vi "play_AFMss_integral_trajTrack_extend.vi"() -> ()   [LabVIEW 2015]
uses:
  controls/controlParams_tracktraj.ctl
  <vilib>/userdefined/High Color/nirio_resource_hc.ctl
  <vilib>/Utility/file.llb/Read From Spreadsheet File (DBL).vi
  <vilib>/FPGAPlugInAG/cRIO-9082/niLvFpga_Open_cRIO-9082.vi
  <vilib>/rvi/interface/common/dynamic/niFpgaDynamicAddResources.vi
  <vilib>/FPGAPlugInAG/Dynamic/niLvFpga_Reset_Dynamic.vi
  <vilib>/rvi/interface/common/niFpgaWaitOnOcc.vi
  <vilib>/Utility/error.llb/Error Cluster From Error Code.vi
  <vilib>/rvi/errors/niLvFpgaAdjustHostInterfaceError.vi
  <vilib>/FPGAPlugInAG/Dynamic/niLvFpga_Run_Dynamic.vi
  <vilib>/Utility/file.llb/Write To Spreadsheet File (DBL).vi
  <vilib>/FPGAPlugInAG/Dynamic/niLvFpga_Close_Dynamic.vi
  <vilib>/rvi/interface/nirviOpenFPGA/nirviOpenFPGA.xnode
  FPGA Bitfiles/AFMsssinglematri_FPGATargetSPARTA_AFMsscontrolDela_G9MTOUg9BHM.lvbitx
  <vilib>/rvi/interface/nirviMethod/nirviMethod.xnode
  <vilib>/rvi/interface/nirviReadWriteControl/nirviReadWriteControl.xnode
  <vilib>/rvi/interface/nirviCloseFPGA/nirviCloseFPGA.xnode
  <vilib>/FPGAPlugInAG/Dynamic/niLvFpga_ConfigureFifo_Dynamic.vi
  <vilib>/rvi/errors/niLvFpgaMergeErrorWithErrorCode.vi
  <vilib>/rvi/interface/Simulation/niFpgaSimulationCallBeginRW.vi
  <vilib>/FPGAPlugInAG/Dynamic/niLvFpga_ReadFifo_Dynamic.vi
  <vilib>/FPGAPlugInAG/Dynamic/niLvFpga_WriteFifo_Dynamic.vi
  NiFpgaLv.dll
panel:
  in  "N":i32
  in  "control_data_path":path=path "C:/Users/arnold/Documents/MATLAB/AFM_SS/data/ref_traj_track.csv"
  out "Actual Depth":u32
  out "YK TO":bool
  out "UK TO":bool
  out "yk":sgl
  out "loop ticks benchmark":sgl
  out "Xd_out(k+1)":sgl[](array[numeric])
  in  "Cluster":T1={"umax"=3.0, "y_ref(k)"=0.0, "Ki"=0.0, "y(k) (from plant)"=0.0, "ND"=0, "NS"=0, "u_Kx_ref(k)"=0.0} {"u_Kx_ref(k)" format="%#_13g"; "Ki" format="%#_13g"; "y_ref(k)" format="%#_13g"; "umax" format="%#_13g"}
  out "Unstable Traj":bool
  out "Control Loop Done":bool
  out "Elements Remaining":u32
  out "Arow10":sgl[](array[numeric])=[0.0, 0.0, 0.0, 0.0, 0.0, 0.0, 0.90156674, 0.0, 0.0]
  out "Arow9":sgl[](array[numeric])=[0.0, 0.0, 0.0, 0.0, 0.0, 0.0, 0.90156674, 0.0, 0.0]
  out "Arow8":sgl[](array[numeric])=[0.0, 0.0, 0.0, 0.0, 0.0, 0.0, 0.90156674, 0.0, 0.0]
  out "elements left":i32=1
  in  "reference traj path":path=path "C:/Users/arnold/Documents/MATLAB/AFM_SS/data/ref_traj_track.csv"
  in  "outputData BOTH":path=path "C:/Users/arnold/Documents/MATLAB/AFM_SS/data/exp01outputBOTH.csv"
  out "x+1":i32
  out "ND":i32
  out "NS":i32
  in  "Tab Control":enum32{"Custom Params", "Loaded Params"}(tab)
  in  "Nbar":dbl=1.253469179440319 format="%#_13g"
  in  "Ki":dbl=0.125346917944 format="%#_13g"
  out "Nbar":dbl=1.253469179440319 format="%#_13g"
  out "Ki":dbl=0.125346917944 format="%#_13g"
  out "ref":dbl format="%#_13g"
  in  "SettleTicks":i32=10
  in  "Stop":bool=TRUE
  out "y iter":i32
  out "u iter":i32
  out "size(s) 5":i32
  out "size(s)":i32
  out "Arow7":sgl[](array[numeric])=[0.0, 0.0, 0.0, 0.0, 0.0, 0.0, 0.90156674, 0.0, 0.0]
  out "Arow6":sgl[](array[numeric])=[0.0, 0.0, 0.0, 0.0, -0.0009308535, 0.009943728, 1.1488396, 0.0, 0.0]
  out "Arow5":sgl[](array[numeric])=[0.0, 0.0, 0.0, 0.0, 0.99437284, 0.09308535, 3.730764, 0.0, 0.0]
  out "Arow4":sgl[](array[numeric])=[0.0, 0.0, -0.16696692, 0.97962993, 29.579603, 1.2871753, 39.36298, 0.0, 0.0]
  out "Arow3":sgl[](array[numeric])=[0.0, 0.0, 0.97962993, 0.16696692, 2.4679432, 0.11174757, 2.9240768, 0.0, 0.0]
  out "K_in 2":sgl[](array[numeric])=[-0.023819132, 0.00010408472, 0.0, 0.0, 0.0, 0.0, 0.0, 0.0, 0.0]
  out "K_in":sgl[](array[numeric])=[-0.023819132, 0.00010408472, 0.0, 0.0, 0.0, 0.0, 0.0, 0.0, 0.0]
  out "Arow2_in":sgl[](array[numeric])=[-0.21879435, 0.97156703, 5.4823804, 0.59487915, 7.8694544, 0.30187303, 8.202156, 0.0, 0.0]
  out "Arow1_in":sgl[](array[numeric])=[0.97156703, 0.21879435, 0.7281903, 0.07828272, 1.117765, 0.037789278, 0.6448556, 0.0, 0.0]
  out "C_in":sgl[](array[numeric])=[-8.076578e-08, -5.6617e-09, 2.3556278e-05, -6.9169624e-07, -0.005420799, 0.00037984832, -0.012524399, 0.0, 0.0]
  out "L_in":sgl[](array[numeric])=[-2254.4756, -17288.861, -3886.0125, -24956.67, -705.887, -3987.6506, -7.2153935, 0.0, 0.0]
  out "Bz_in":sgl[](array[numeric])=[-0.0016434871, -0.020676594, -0.010679029, -0.20639984, -0.030792456, -1.3413852, -0.02736353, 0.0, 0.0]
  in  "Iters":i32=25
  in  "Cont Run (F)":bool=TRUE
  in  "ymax":dbl=4.0 format="%#_13g"
  in  "umax":dbl=1.0 format="%#_13g"
  in  "TsTicks":i32=1600
  # "Manually define Parameters"
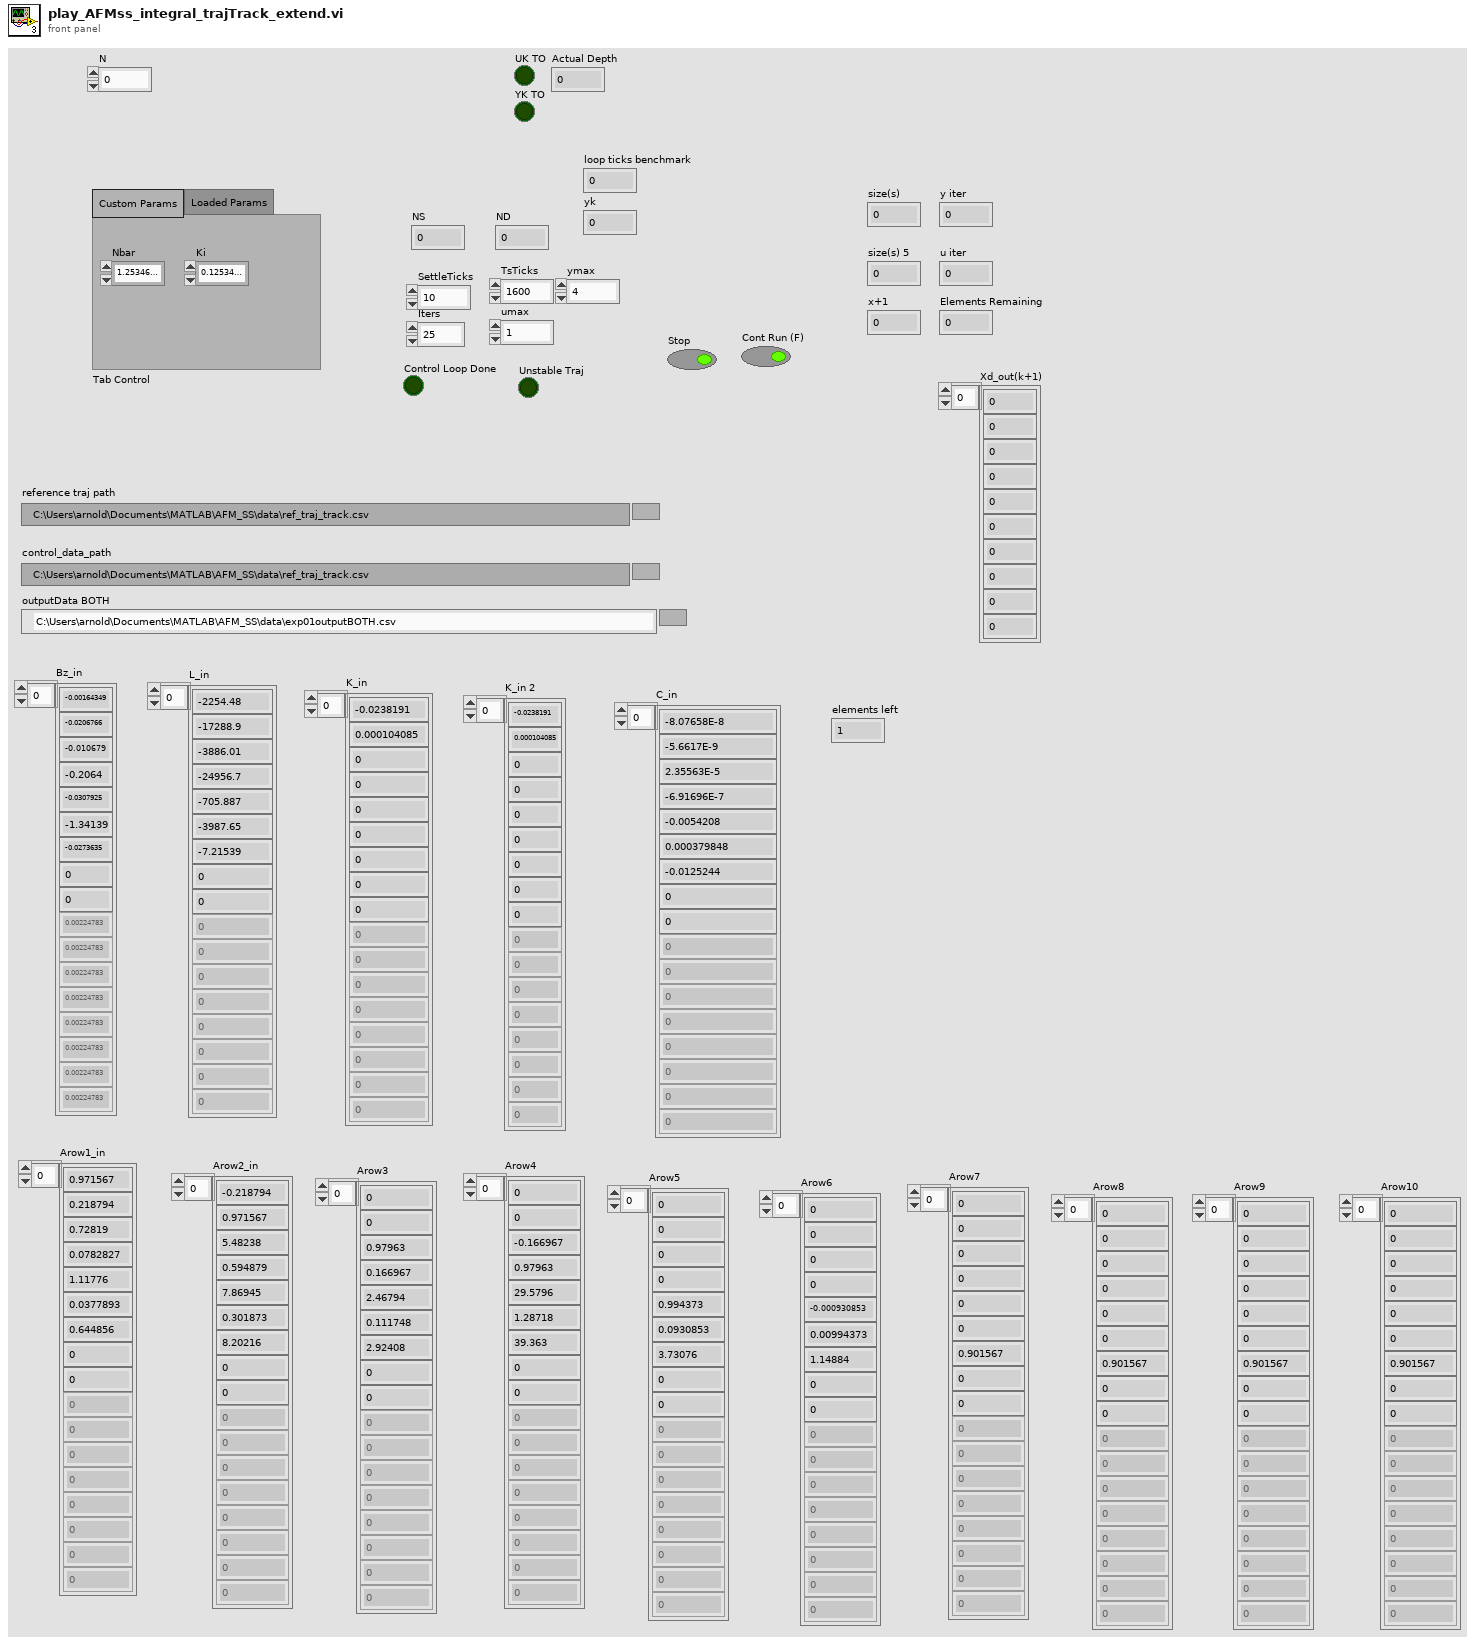
[diagram p1: front panel]
types:
  T1 = typedef "controlParams_tracktraj.ctl" = cluster{"umax":sgl, "y_ref(k)":sgl, "Ki":sgl, "y(k) (from plant)":sgl, "ND":i16, "NS":i16, "u_Kx_ref(k)":sgl}
  T2 = typedef "nirio_resource_hc.ctl" = tag
  T3 = typedef "ControlParams.ctl" = cluster{"NS":i32, "ND":i32, "Nbar":dbl, "Ki":dbl, "ref":dbl}
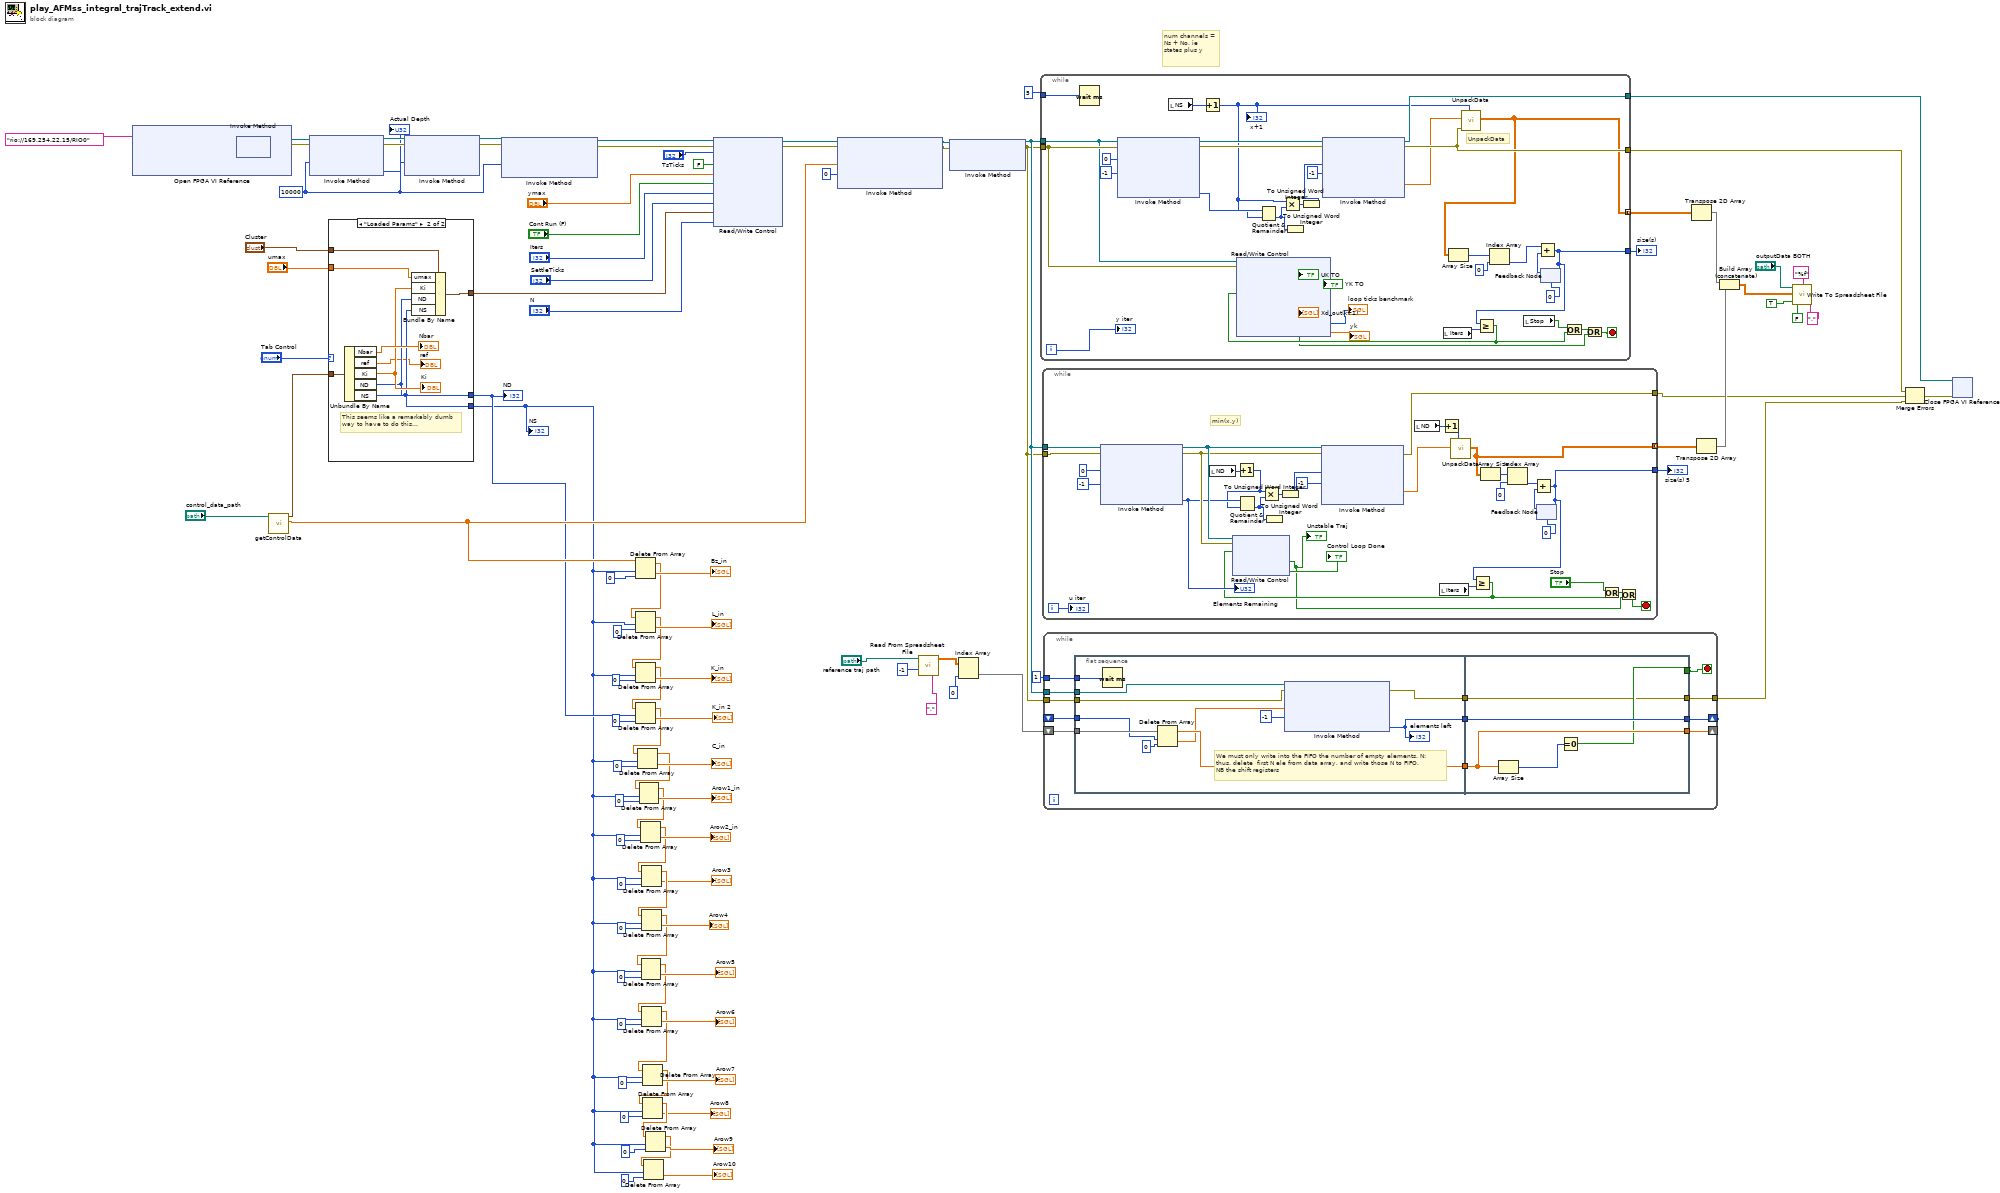
[diagram p0: block diagram]
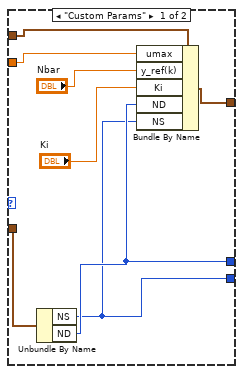
[diagram p2: hidden frame]
diagram:
  w46 = 10000
  # "num channels = Ns + No, ie states plus y"
  n1 = xnode "Open FPGA VI Reference"("resource name"=T2 "rio://169.254.22.15/RIO0") -> ("FPGA VI Reference Out"=w41:refnum<k20>, "error out"=w40:errorcluster)  [unwired: 1 in]
  n2 = xnode "Invoke Method"("FPGA VI Reference In"=w41, "error in"=w40) -> ("FPGA VI Reference Out"=w53:refnum<k20>, "error out"=w52:errorcluster)
  n3 = call "getControlData.vi"("system matricec path"="control_data_path") -> ("AllMatrix"=w45:dbl[], "controlParams"=w44:T3)  [unwired: 9 in]
  n4 = xnode "Invoke Method"("FPGA VI Reference In"=w53, "error in"=w52, "Requested Depth"=w46) -> ("FPGA VI Reference Out"=w105:refnum<k20>, "error out"=w104:errorcluster, "Actual Depth"=→"Actual Depth":u32)
  n5 = case shown="\"Loaded Params\"" "Tab Control" {
    tunnel: w44 -> [w113 w122]
    tunnel: [w107 w117] -> w11
    tunnel: [w108 w118] -> w42
    tunnel: "umax" -> [w112 w115]
    tunnel: [w110 w119] -> w8
    tunnel: "Cluster" -> [w106 w116]
    frame "Custom Params" {
      n6 = Unbundle By Name(w113) -> ("NS"=w107:i32, "ND"=w108:i32)
      n7 = Bundle By Name(cluster=w106, "umax"=w112, "y_ref(k)"="Nbar", "Ki"="Ki", "ND"=w108, "NS"=w107) -> (w110:T1)
    }
    frame "Loaded Params" {
      # "This seems like a remarkably dumb\nway to have to do this..."
      n8 = Unbundle By Name(w122) -> ("Nbar"=→"Nbar":dbl, "ref"=→"ref":dbl, "Ki"=w120:dbl, "ND"=w118:i32, "NS"=w117:i32)
      "Ki" <- w120
      n9 = Bundle By Name(cluster=w116, "umax"=w115, "Ki"=w120, "ND"=w118, "NS"=w117) -> (w119:T1)
    }
  }
  "NS" <- w11
  "ND" <- w42
  n10 = xnode "Invoke Method"("FPGA VI Reference In"=w105, "error in"=w104, "Requested Depth"=w46) -> ("FPGA VI Reference Out"=w50:refnum<k20>, "error out"=w49:errorcluster)  [unwired: 1 out]
  n11 = xnode "Invoke Method"("FPGA VI Reference In"=w50, "error in"=w49, "Requested Depth"=w46) -> ("FPGA VI Reference Out"=w48:refnum<k20>, "error out"=w47:errorcluster)  [unwired: 1 out]
  n12 = Delete From Array(array=w45, length=w11, index=0) -> (deleted portion=→"Bz_in":dbl[], array with subset deleted=w89:dbl[])
  n13 = Delete From Array(array=w89, length=w11, index=0) -> (deleted portion=→"L_in":dbl[], array with subset deleted=w86:dbl[])
  n14 = Delete From Array(array=w86, length=w11, index=0) -> (deleted portion=→"K_in":dbl[], array with subset deleted=w82:dbl[])
  n15 = Delete From Array(array=w82, length=w42, index=0) -> (deleted portion=→"K_in 2":dbl[], array with subset deleted=w79:dbl[])
  n16 = Delete From Array(array=w79, length=w11, index=0) -> (deleted portion=→"C_in":dbl[], array with subset deleted=w76:dbl[])
  n17 = Delete From Array(array=w76, length=w11, index=0) -> (deleted portion=→"Arow1_in":dbl[], array with subset deleted=w73:dbl[])
  n18 = Delete From Array(array=w73, length=w11, index=0) -> (deleted portion=→"Arow2_in":dbl[], array with subset deleted=w66:dbl[])
  n19 = Delete From Array(array=w66, length=w11, index=0) -> (deleted portion=→"Arow3":dbl[], array with subset deleted=w65:dbl[])
  n20 = Delete From Array(array=w65, length=w11, index=0) -> (deleted portion=→"Arow4":dbl[], array with subset deleted=w62:dbl[])
  n21 = Delete From Array(array=w62, length=w11, index=0) -> (deleted portion=→"Arow5":dbl[], array with subset deleted=w60:dbl[])
  n22 = Delete From Array(array=w60, length=w11, index=0) -> (deleted portion=→"Arow6":dbl[], array with subset deleted=w58:dbl[])
  n23 = Delete From Array(array=w58, length=w11, index=0) -> (deleted portion=→"Arow7":dbl[], array with subset deleted=w18:dbl[])
  n24 = Delete From Array(array=w18, length=w11, index=0) -> (deleted portion=→"Arow8":dbl[], array with subset deleted=w16:dbl[])
  n25 = Delete From Array(array=w16, length=w11, index=0) -> (deleted portion=→"Arow9":dbl[], array with subset deleted=w12:dbl[])
  n26 = Delete From Array(array=w12, length=w11, index=0) -> (deleted portion=→"Arow10":dbl[])  [unwired: 1 out]
  n27 = xnode "Read/Write Control"("FPGA VI Reference In"=w48, "error in"=w47, "TsTicks"="TsTicks", "Abort"=FALSE, "ymax"="ymax", "False  = cont run"="Cont Run (F)", "iters"="Iters", "Settle Ticks"="SettleTicks", "Cluster"=w8, "N"="N") -> ("FPGA VI Reference Out"=w94:refnum<k20>, "error out"=w93:errorcluster)
  n28 = xnode "Invoke Method"("FPGA VI Reference In"=w94, "error in"=w93, "Data"=w45, "Timeout (ms)"=0) -> ("FPGA VI Reference Out"=w97:refnum<k20>, "error out"=w96:errorcluster)  [unwired: 1 out]
  n29 = call-poly <vilib>:"Read From Spreadsheet File.vi"("delimiter (\\t)"=",", "number of rows (all:-1)"=-1, "file path (dialog if empty)"="reference traj path") -> ("all rows"=w25:dbl[][])  [unwired: 4 in, 4 out]
  n30 = xnode "Invoke Method"("FPGA VI Reference In"=w97, "error in"=w96) -> ("FPGA VI Reference Out"=w6:refnum<k20>, "error out"=w5:errorcluster)  [unwired: 1 in]
  n31 = Index Array(array=w25, index (col)=0 ("dimension size")) -> (element=w23:dbl[])  [unwired: 1 in]
  n32 = while {
    tunnel: 5 -> [w158]
    tunnel: w6 -> [w136]
    tunnel: w5 -> [w137]
    tunnel: [w150] -> w22
    tunnel: [w149] -> w92
    tunnel: [w135] -> w56 mode=concatenating
    tunnel: [w133] -> w54
    i -> [w134]
    stop <- w128 stop-if-true
    # "UnpackData"
    n33 = Wait (ms)(milliseconds to wait=w158) -> ()  [unwired: 1 out]
    n34 = xnode "Invoke Method"("FPGA VI Reference In"=w136, "error in"=w137, "Number of Elements"=0 ("Timeout (ms)"), "Timeout (ms)"=-1) -> ("FPGA VI Reference Out"=w154:refnum<k20>, "error out"=w155:errorcluster, "Elements Remaining"=w145:u32)  [unwired: 1 out]
    n35 = local read "NS"() -> (w144:i32)
    n36 = Increment(x=w144) -> (x+1=w143:i32)
    "x+1" <- w143
    n37 = Quotient & Remainder(x=w145, y=w143) -> (floor(x/y)=w147:u32)  [unwired: 1 out]
    n38 = Multiply(x=w143, y=w147) -> (x*y=w152:u32)
    n39 = To Unsigned Word Integer(number=w147) -> ()  [unwired: 1 out]
    n40 = To Unsigned Word Integer(number=w152) -> (unsigned 16bit integer=w148:u16)
    n41 = xnode "Invoke Method"("FPGA VI Reference In"=w154, "error in"=w155, "Number of Elements"=w148, "Timeout (ms)"=-1) -> ("FPGA VI Reference Out"=w149:refnum<k20>, "error out"=w150:errorcluster, "Data"=w142:sgl[])  [unwired: 1 out]
    n42 = local read "Iters"() -> (w146:i32)
    n43 = call "UnpackData.vi"("NumChannels"=w143, "error In"=w150, "1D Data In"=w142) -> ("2D Data Out"=w135:dbl[][])  [unwired: 7 in, 1 out]
    n44 = Array Size(array=w135) -> (size(s)=w141:i32[])
    n45 = Index Array(array=w141, index=0) -> (element=w139:i32)
    n46 = local read "Stop"() -> (w131:bool)
    n47 = feedback #1(0) -> (w140:i32)
    n48 = Add(x=w139, y=w140) -> (x+y=w133:i32)
    n49 = Greater Or Equal?(x=w133, y=w146) -> (x >= y?=w132:bool)
    n50 = xnode "Read/Write Control"("FPGA VI Reference In"=w136, "error in"=w137, "Abort"=w132) -> ("UK TO"=→"UK TO":bool, "YK TO"=→"YK TO":bool, "Unstable Traj"=w129:bool, "Xd_out(k+1)"=→"Xd_out(k+1)":sgl[], "Loop Ticks (benchmark)"=→"loop ticks benchmark":i16, "yk"=→"yk":sgl)  [unwired: 2 out]
    n51 = feedback-in #1(w133) -> ()
    n52 = Or(x=w131, y=w132) -> (x .or. y?=w130:bool)
    n53 = Or(x=w130, y=w129) -> (x .or. y?=w128:bool)
    "y iter" <- w134
  }
  "size(s)" <- w54
  n54 = while {
    tunnel: [w167] -> w43 mode=concatenating
    tunnel: w6 -> [w177]
    tunnel: w5 -> [w176]
    tunnel: [w174] -> w55
    tunnel: [w163] -> w20
    i -> [w175]
    stop <- w162 stop-if-true
    # "min(x,y)"
    n55 = xnode "Invoke Method"("FPGA VI Reference In"=w177, "error in"=w176, "Number of Elements"=0 ("Timeout (ms)"), "Timeout (ms)"=-1) -> ("FPGA VI Reference Out"=w185:refnum<k20>, "error out"=w184:errorcluster, "Elements Remaining"=w181:u32)  [unwired: 1 out]
    "Elements Remaining" <- w181
    n56 = local read "ND"() -> (w170:i32)
    n57 = Increment(x=w170) -> (x+1=w179:i32)
    n58 = Quotient & Remainder(x=w181, y=w179) -> (floor(x/y)=w182:u32)  [unwired: 1 out]
    n59 = Multiply(x=w179, y=w182) -> (x*y=w183:u32)
    n60 = To Unsigned Word Integer(number=w182) -> ()  [unwired: 1 out]
    n61 = To Unsigned Word Integer(number=w183) -> (unsigned 16bit integer=w180:u16)
    n62 = xnode "Invoke Method"("FPGA VI Reference In"=w185, "error in"=w184, "Number of Elements"=w180, "Timeout (ms)"=-1) -> ("error out"=w163:errorcluster, "Data"=w171:sgl[])  [unwired: 2 out]
    n63 = local read "ND"() -> (w169:i32)
    n64 = local read "Iters"() -> (w186:i32)
    n65 = Increment(x=w169) -> (x+1=w166:i32)
    n66 = call "UnpackData.vi"("NumChannels"=w166, "1D Data In"=w171) -> ("2D Data Out"=w167:dbl[][])  [unwired: 8 in, 1 out]
    n67 = Array Size(array=w167) -> (size(s)=w164:i32[])
    n68 = Index Array(array=w164, index=0) -> (element=w168:i32)
    n69 = feedback #2(0) -> (w178:i32)
    n70 = Add(x=w168, y=w178) -> (x+y=w174:i32)
    n71 = Greater Or Equal?(x=w174, y=w186) -> (x >= y?=w173:bool)
    n72 = xnode "Read/Write Control"("FPGA VI Reference In"=w185, "error in"=w184, "Abort"=w173) -> ("Unstable Traj"=w159:bool, "Loop Done"=→"Control Loop Done":bool)  [unwired: 2 out]
    "Unstable Traj" <- w159
    n73 = feedback-in #2(w174) -> ()
    n74 = Or(x="Stop", y=w173) -> (x .or. y?=w161:bool)
    n75 = Or(x=w161, y=w159) -> (x .or. y?=w162:bool)
    "u iter" <- w175
  }
  "size(s) 5" <- w55
  n76 = while {
    tunnel: [w200] -> w19
    tunnel: 1 -> [w202]
    shift-right: [w195] -> _
    shift-left: _ -> [w199]
    shift-right: [w193] -> _
    shift-left: w23 -> [w201]
    tunnel: w6 -> [w192]
    tunnel: w5 -> [w191]
    stop <- w196 stop-if-true
    n77 = flat-sequence {
      tunnel: w202 -> [w213]
      tunnel: w201 -> [w208]
      tunnel: w199 -> [w204]
      tunnel: [w211] -> w198
      tunnel: [w209] -> w197
      tunnel: [w210] -> w194
      tunnel: w192 -> [w206]
      tunnel: w191 -> [w205]
      tunnel: [w218] -> w195
      tunnel: [w214] -> w200
      tunnel: w198 -> [w214]
      tunnel: w197 -> [w218]
      tunnel: [w215] -> w196
      tunnel: w194 -> [w216]
      tunnel: [w216] -> w193
      frame #0 {
        # "We must only write into the FIFO the number of empty elements, N:\nthus, delete  first N ele from data array, and write those N to FIFO.\nNB the shift registers"
        n78 = Wait (ms)(milliseconds to wait=w213) -> ()  [unwired: 1 out]
        n79 = Delete From Array(array=w208, length=w204, index=0) -> (deleted portion=w207:dbl[], array with subset deleted=w210:dbl[])
        n80 = xnode "Invoke Method"("FPGA VI Reference In"=w206, "error in"=w205, "Data"=w207, "Timeout (ms)"=-1) -> ("error out"=w211:errorcluster, "Empty Elements Remaining"=w209:u32)  [unwired: 1 out]
        "elements left" <- w209
      }
      frame #1 {
        n81 = Array Size(array=w216) -> (size(s)=w217:i32)
        n82 = Equal To 0?(x=w217) -> (x = 0?=w215:bool)
      }
    }
  }
  n83 = Transpose 2D Array(2D array=w56) -> (transposed array=w37:dbl[][])
  n84 = Transpose 2D Array(2D array=w43) -> (transposed array=w36:dbl[][])
  n85 = Build Array (concatenate)(w37, w36) -> (w30:dbl[][])
  n86 = call-poly <vilib>:"Write To Spreadsheet File.vi"("delimiter (\\t)"=",", "transpose? (no:F)"=TRUE, "format (%.3f)"="%f", "append to file? (new file:F)"=FALSE, "2D data"=w30, "file path (dialog if empty)"="outputData BOTH") -> ()  [unwired: 2 in, 1 out]
  n87 = Merge Errors(w22, w20, w19) -> (w21:errorcluster)
  n88 = xnode "Close FPGA VI Reference"("FPGA VI Reference In"=w92, "error in"=w21) -> ()  [unwired: 1 out]
